vi "EFMC-SET-1.vi"(4 "气压高度数据有效性":refnum<vi>, 5 "GNSS1卫星禁用控制字":refnum<vi>, 6 "组合模式控制字":refnum<vi>, 7 "GNSS2卫星禁用控制字":refnum<vi>, 9 "组合模式":refnum<vi>, 10 "GNSS3卫星禁用控制字":refnum<vi>, 11 "气压高度":refnum<vi>) -> (3 "添加的数组":u8[](array[numeric]))   [LabVIEW 2012]
uses:
  XX-I32.vi
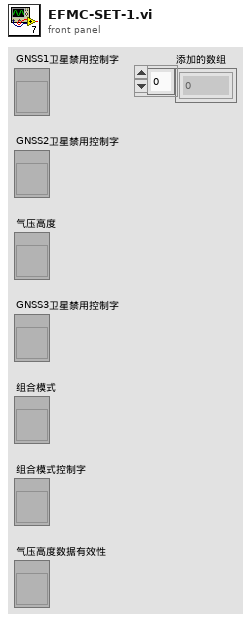
[diagram p1: front panel]
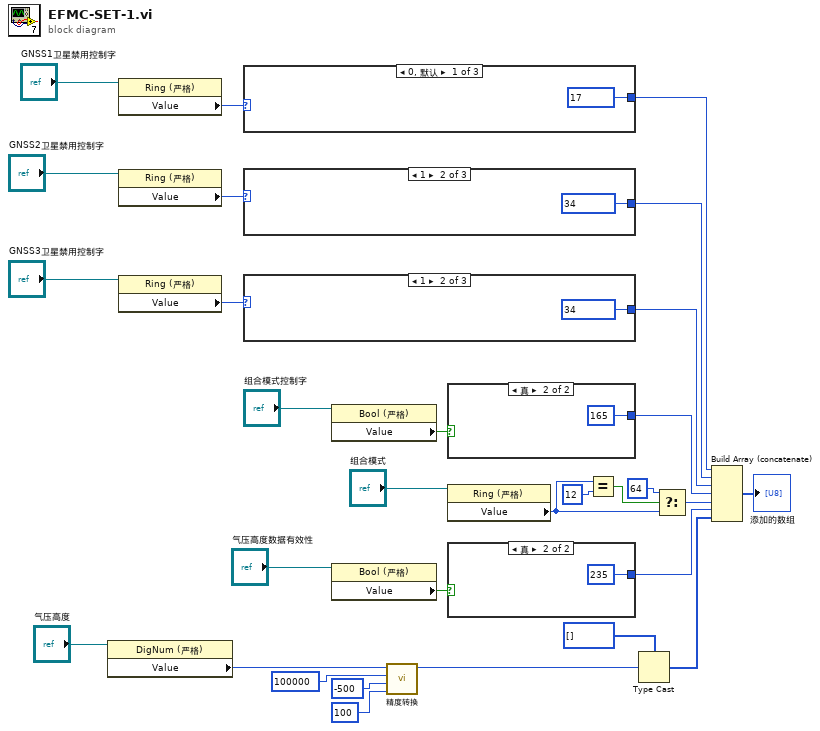
[diagram p0: block diagram]
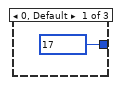
[diagram p4: hidden frame]
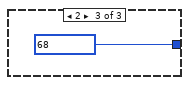
[diagram p5: hidden frame]
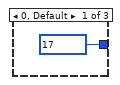
[diagram p6: hidden frame]
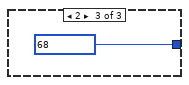
[diagram p7: hidden frame]
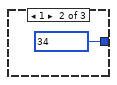
[diagram p8: hidden frame]
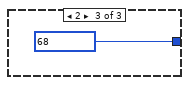
[diagram p9: hidden frame]
diagram:
  n1 = property on="属性节点" class="DigNum (严格)"(reference="气压高度") -> ("Value"=w27:i32)  [unwired: 1 in, 2 out]
  n2 = property on="属性节点" class="Ring (严格)"(reference="GNSS1卫星禁用控制字") -> ("Value"=w8:u8)  [unwired: 1 in, 2 out]
  n3 = property on="属性节点" class="Ring (严格)"(reference="GNSS2卫星禁用控制字") -> ("Value"=w10:u8)  [unwired: 1 in, 2 out]
  n4 = property on="属性节点" class="Ring (严格)"(reference="GNSS3卫星禁用控制字") -> ("Value"=w12:u8)  [unwired: 1 in, 2 out]
  n5 = case shown="0, 默认" w8 {
    tunnel: [u8 17 u8 34 u8 68] -> w9
    frame 0, Default {
    }
    frame 1 {
    }
    frame 2 {
    }
  }
  n6 = case shown="1" w10 {
    tunnel: [u8 17 u8 34 u8 68] -> w11
    frame 0, Default {
    }
    frame 1 {
    }
    frame 2 {
    }
  }
  n7 = case shown="1" w12 {
    tunnel: [u8 17 u8 34 u8 68] -> w13
    frame 0, Default {
    }
    frame 1 {
    }
    frame 2 {
    }
  }
  n8 = property on="属性节点" class="Bool (严格)"(reference="组合模式控制字") -> ("Value"=w14:bool)  [unwired: 1 in, 2 out]
  n9 = property on="属性节点" class="Bool (严格)"(reference="气压高度数据有效性") -> ("Value"=w21:bool)  [unwired: 1 in, 2 out]
  n10 = call-poly "精度转换.vi"("单位"=100, "下限"=-500, "上限"=100000, "数值输入"=w27) -> ("输出"=w25:i32)  [unwired: 7 in]
  n11 = case shown="真" w14 {
    tunnel: [_ u8 165] -> w15
    frame False {
    }
    frame True {
    }
  }
  n12 = property on="属性节点" class="Ring (严格)"(reference="组合模式") -> ("Value"=w19:u8)  [unwired: 1 in, 2 out]
  n13 = case shown="真" w21 {
    tunnel: [_ u8 235] -> w22
    frame False {
    }
    frame True {
    }
  }
  n14 = Equal?(x=w19, y=u8 12) -> (x = y?=w17:bool)
  n15 = Type Cast(type=u8[] [], x=w25) -> (*(type *) &x=w29:u8[])
  n16 = Select(t=u8 64, s=w17, f=w19) -> (s? t:f=w20:u8)
  n17 = Build Array (concatenate)(w9, w11, w13, w15, w20, w22, w29) -> (→"添加的数组":u8[])
